vi "Normalized Range Compare.vi"(2 "Y Averages":dbl[](graph), 3 "X Averages":dbl[](graph)) -> (0 "Y Score":dbl, 1 "X Score":dbl)   [LabVIEW 2012]
doc: "The input data represents the average pixels set for each row and each column of the possible target. Since targets are expected to have a hollow center, compare the pixel averages to the expected min and max values across the target. Higher scores indicate a strong border and hollow center."
panel:
  out "XY Graph":cluster{"Y Averages":dbl[], i32[]}[](graph)
  in  "Y Min":dbl[](array[numeric])=[0.4, 0.6, 0.05, 0.05, 0.05, 0.05, 0.05, 0.05, 0.05, 0.05, 0.05, 0.05, 0.05, 0.05, 0.05, 0.05, 0.05, 0.05, 0.05, 0.05, 0.05, 0.05, 0.05, 0.05, 0.05, 0.05, 0.05, 0.05, 0.05, 0.05, 0.05, 0.05, 0.05, 0.05, 0.05, 0.05, 0.05, 0.05, 0.05, 0.05, 0.05, 0.05, 0.05, 0.05, 0.05, 0.05, 0.6, 0.0]
  in  "Y Max":dbl[](array[numeric])=[1.0, 1.0, 1.0, 1.0, 0.5, 0.5, 0.5, 0.5, 0.5, 0.5, 0.5, 0.5, 0.5, 0.5, 0.5, 0.5, 0.5, 0.5, 0.5, 0.5, 1.0, 1.0, 1.0, 1.0]
  in  "X Min":dbl[](array[numeric])=[0.4, 0.6, 0.1, 0.1, 0.1, 0.1, 0.1, 0.1, 0.1, 0.1, 0.1, 0.1, 0.1, 0.1, 0.1, 0.1, 0.1, 0.1, 0.1, 0.1, 0.1, 0.1, 0.6, 0.0]
  out "X Results":dbl[][](graph)
  in  "X Max":dbl[](array[numeric])=[1.0, 1.0, 1.0, 1.0, 0.5, 0.5, 0.5, 0.5, 0.5, 0.5, 0.5, 0.5, 0.5, 0.5, 0.5, 0.5, 0.5, 0.5, 0.5, 0.5, 1.0, 1.0, 1.0, 1.0]
  # "Measure the values against the scaled values, counting how many are between the min and max."
  # "Flipped"
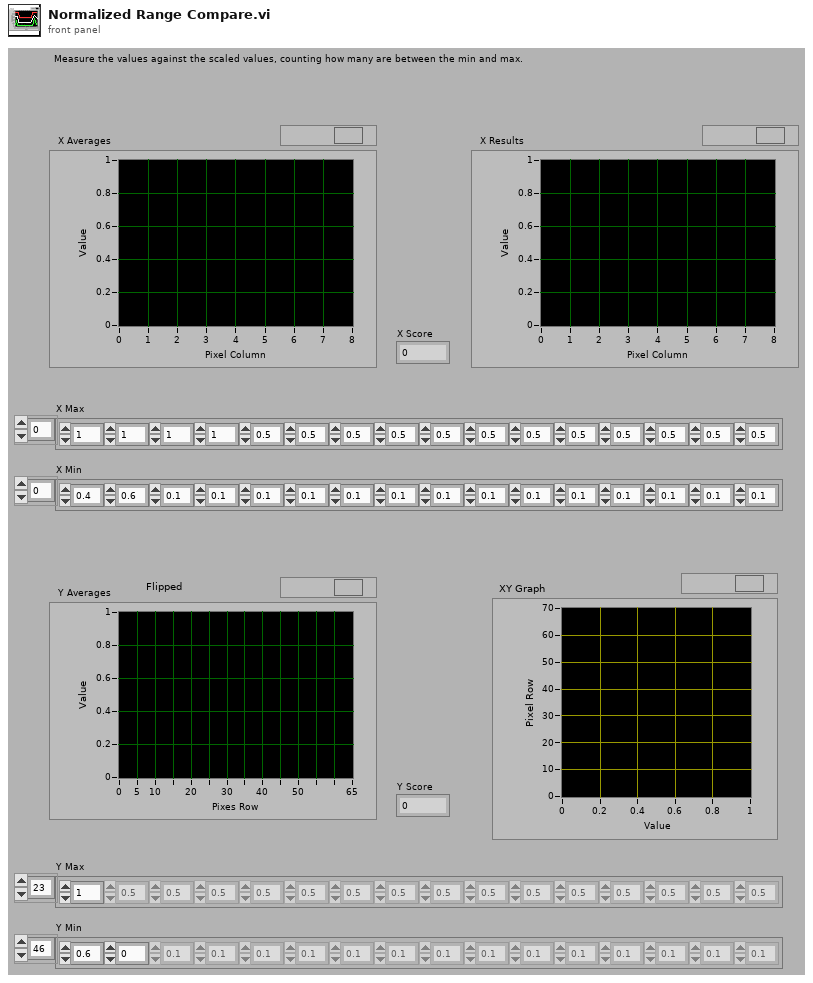
[diagram p1: front panel]
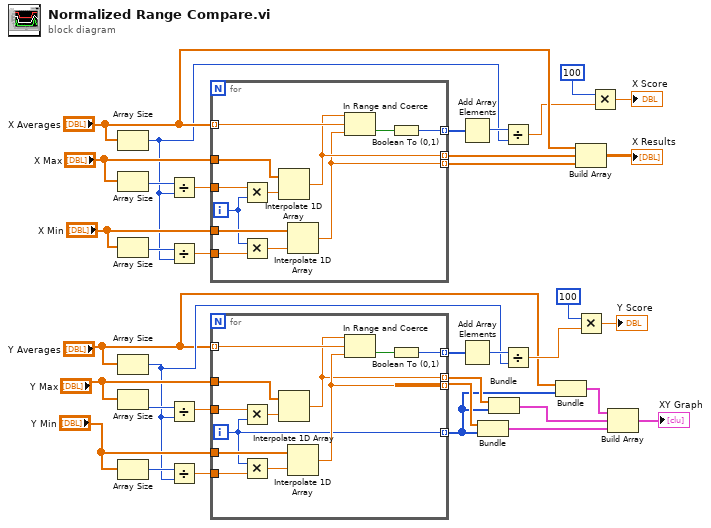
[diagram p0: block diagram]
diagram:
  n1 = Array Size(array="X Averages") -> (size(s)=w16:i32)
  n2 = Array Size(array="X Max") -> (size(s)=w31:i32)
  n3 = Array Size(array="X Min") -> (size(s)=w24:i32)
  n4 = Array Size(array="Y Averages") -> (size(s)=w15:i32)
  n5 = Array Size(array="Y Max") -> (size(s)=w29:i32)
  n6 = Array Size(array="Y Min") -> (size(s)=w26:i32)
  n7 = Divide(x=w31, y=w16) -> (x/y=w30:dbl)
  n8 = Divide(x=w24, y=w16) -> (x/y=w22:dbl)
  n9 = Divide(x=w29, y=w15) -> (x/y=w27:dbl)
  n10 = Divide(x=w26, y=w15) -> (x/y=w21:dbl)
  n11 = for {
    tunnel: "X Averages" -> [w48] mode=indexing
    tunnel: "X Max" -> [w46]
    tunnel: [w45] -> w36 mode=indexing
    tunnel: [w42] -> w35 mode=indexing
    tunnel: w30 -> [w47]
    tunnel: "X Min" -> [w44]
    tunnel: w22 -> [w40]
    tunnel: [w37] -> w20 mode=indexing
    i -> [w41]
    n12 = Multiply(x=w47, y=w41) -> (x*y=w43:dbl)
    n13 = Multiply(x=w41, y=w40) -> (x*y=w39:dbl)
    n14 = Interpolate 1D Array(1:w43, 2:w46) -> (0:w45:dbl)
    n15 = Interpolate 1D Array(1:w39, 2:w44) -> (0:w42:dbl)
    n16 = In Range and Coerce(upper limit=w45, x=w48, lower limit=w42) -> (In Range?=w38:bool)  [unwired: 1 out]
    n17 = Boolean To (0,1)(Boolean=w38) -> (0, 1=w37:i16)
  }
  n18 = for {
    tunnel: "Y Averages" -> [w60] mode=indexing
    tunnel: "Y Max" -> [w58]
    tunnel: [w50] -> w6 mode=indexing
    tunnel: [w51] -> w8 mode=indexing
    tunnel: w27 -> [w59]
    tunnel: "Y Min" -> [w57]
    tunnel: w21 -> [w54]
    tunnel: [w52] -> w19 mode=indexing
    tunnel: [w49] -> w3 mode=indexing
    i -> [w49]
    n19 = Multiply(x=w59, y=w49) -> (x*y=w56:dbl)
    n20 = Multiply(x=w49, y=w54) -> (x*y=w55:dbl)
    n21 = Interpolate 1D Array(1:w56, 2:w58) -> (0:w50:dbl)
    n22 = Interpolate 1D Array(1:w55, 2:w57) -> (0:w51:dbl)
    n23 = In Range and Coerce(upper limit=w50, x=w60, lower limit=w51) -> (In Range?=w53:bool)  [unwired: 1 out]
    n24 = Boolean To (0,1)(Boolean=w53) -> (0, 1=w52:i16)
  }
  n25 = Add Array Elements(numeric array=w20) -> (sum=w17:i16)
  n26 = Add Array Elements(numeric array=w19) -> (sum=w18:i16)
  n27 = Bundle(w8, w3) -> (w7:cluster{dbl[], i32[]})  [unwired: 1 in]
  n28 = Bundle(w6, w3) -> (w5:cluster{dbl[], i32[]})  [unwired: 1 in]
  n29 = Divide(x=w17, y=w16) -> (x/y=w14:dbl)
  n30 = Divide(x=w18, y=w15) -> (x/y=w11:dbl)
  n31 = Bundle("Y Averages"="Y Averages", w3) -> (w2:cluster{"Y Averages":dbl[], i32[]})  [unwired: 1 in]
  n32 = Build Array("X Averages", w36, w35) -> (→"X Results":dbl[][])
  n33 = Multiply(x=100, y=w11) -> (x*y=→"Y Score":dbl)
  n34 = Multiply(x=100, y=w14) -> (x*y=→"X Score":dbl)
  n35 = Build Array(w2, w5, w7) -> (→"XY Graph":cluster{"Y Averages":dbl[], i32[]}[])
